vi "tester.vi"   [LabVIEW 2020, in "Method Generation.lvlib" / "New Setter Dialog.lvclass"]
uses:
  New Setter Dialog.lvclass
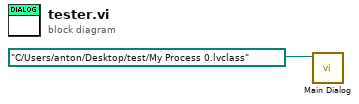
[diagram p0: block diagram]
diagram:
  n1 = call "Main Dialog.vi"("Process Path"=path "C:/Users/anton/Desktop/test/My Process 0.lvclass" ("class path")) -> ()  [unwired: 11 in]
